vi "Actor Core.vi"(8 "error in":errorcluster, 11 "Preview in":refnum<class "Preview.lvclass">) -> (0 "error out":errorcluster, 3 "Actor out":refnum<class "Actor.lvclass">)   [LabVIEW 2018, in "Preview Window.lvlib" / "Preview.lvclass"]
doc: "(<B>Filename</B>: Actor Framework.lvlib:Actor.lvclass:Actor Core.vi)\n\nReceives messages to the actor, reacts to them, and initiates any error handling that may shut the actor down.\n\nDescendant classes may override this VI to append parallel tasks for the actor to complete while it handles messages. Overrides use the Call Parent Method node."
uses:
  Preview.lvclass
  C:/Users/Jeff Tipps/Documents/DAQMan/source/Classes/Actor Nest/Class Actor Nest/Actor Nest.lvclass
  C:/Program Files (x86)/National Instruments/LabVIEW 2018/vi.lib/ActorFramework/Actor/Actor.lvclass
  <vilib>/ActorFramework/Actor/Actor.lvclass
  Actor Nest/Class Actor Nest/Actor Nest.lvclass/Actor Nest.ctl
  <vilib>/ActorFramework/Actor/Actor.lvclass/Actor.ctl
  <vilib>/ActorFramework/Message Enqueuer/Message Enqueuer.lvclass/Message Enqueuer.ctl
  Actor Nest/Actor Nest Messages/Handle Nested Error Msg/Handle Nested Error Msg.lvclass/Handle Nested Error Msg.ctl
  Actor Nest/Class Actor Nest/Read Shutdown.vi
  <vilib>/ActorFramework/Message Enqueuer/Init from Existing Queue.vi
  <vilib>/ActorFramework/Message Enqueuer/Enqueue.vi
  Actor Nest/Actor Nest Messages/Handle Nested Error Msg/Handle Nested Error Msg.lvclass
  C:/Program Files (x86)/National Instruments/LabVIEW 2018/vi.lib/ActorFramework/Message/Message.lvclass
  <vilib>/ActorFramework/Stop Msg/Stop Msg.lvclass
  <vilib>/ActorFramework/Message Priority Queue/Priority Enqueue.vi
  <vilib>/ActorFramework/Message Enqueuer/Message Enqueuer.lvclass
  Actor Nest/Class Actor Nest/Actor Nest.lvclass
panel:
  in  "Stop Scalar":bool
  in  "Stop Wfm":bool
  in  "Legend LB":i32[](listbox)
  out "Wfm Graph":sgl[][](graph)
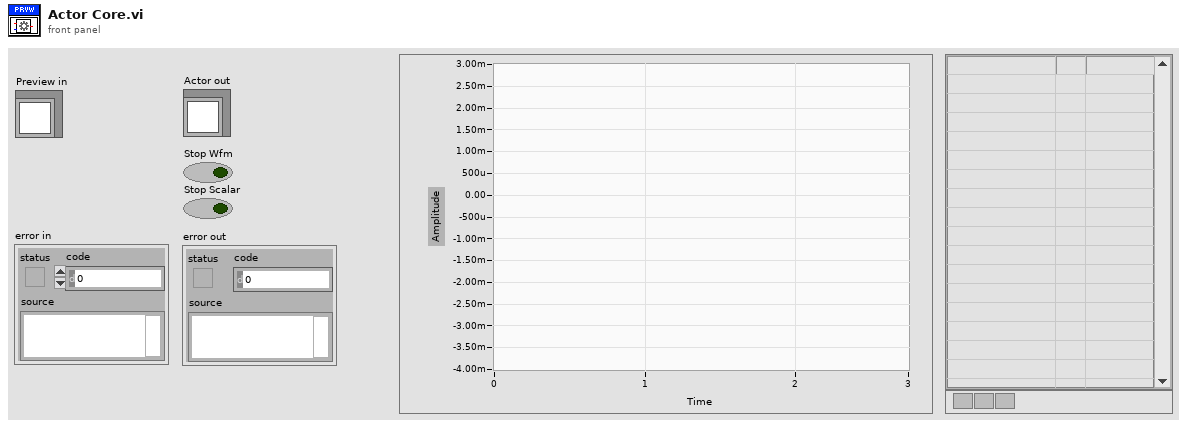
[diagram p1: front panel]
types:
  T1 = cluster{"Scalar Ntfr Name":string, "Num of Chans":i32, "Selected Chan Indeces":i32[]}
  T2 = cluster{"Wfm Ntfr Name":string, "Chart History":i32, "Selected Chan Indeces":i32[]}
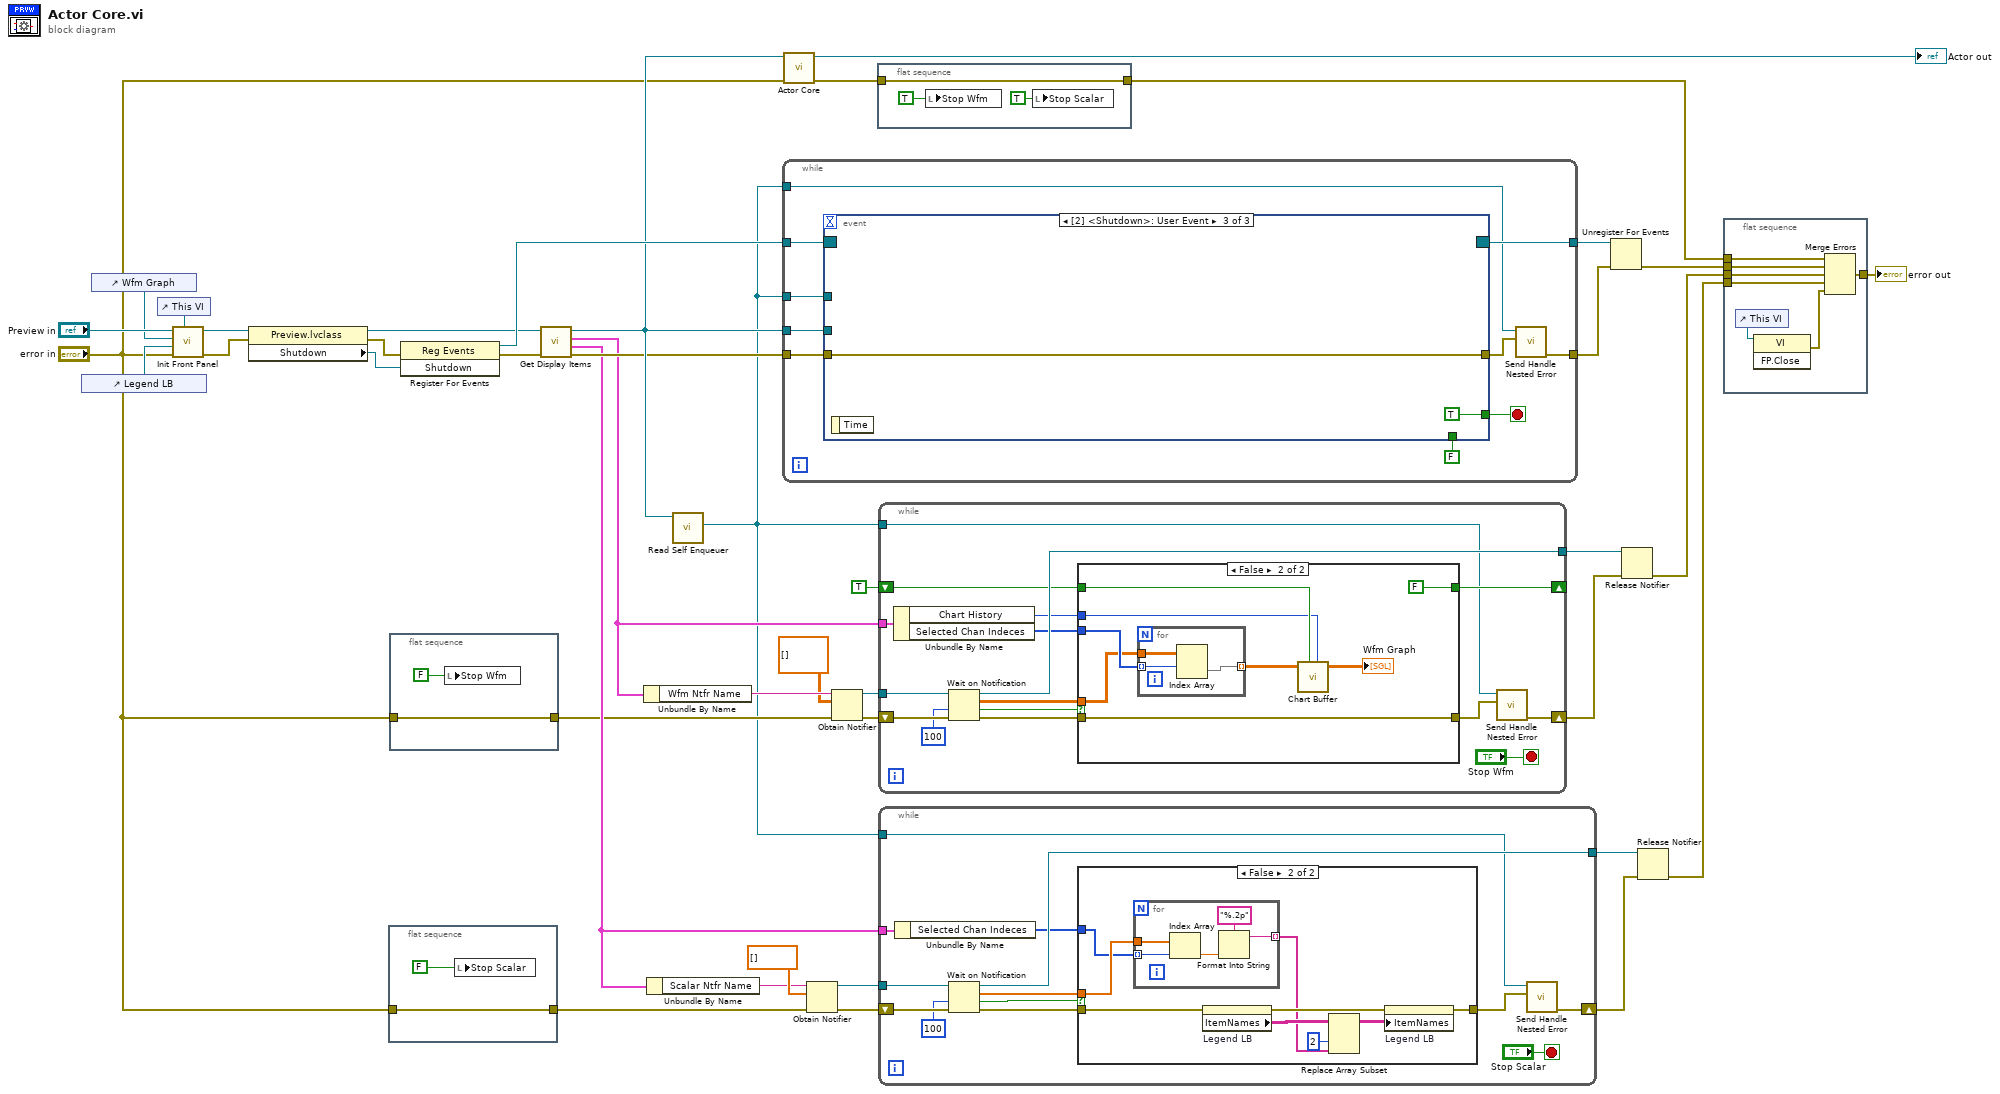
[diagram p0: block diagram]
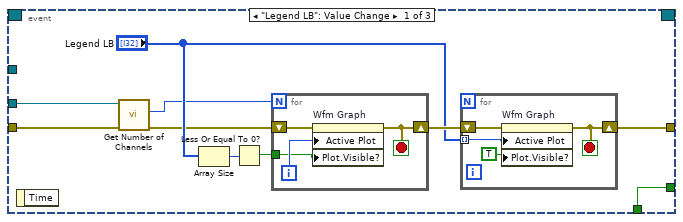
[diagram p4: hidden frame]
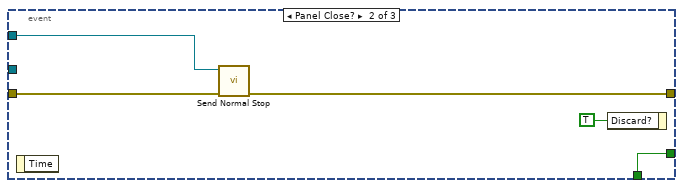
[diagram p5: hidden frame]
diagram:
  n1 = control-ref of="Legend LB"() -> (w40:refnum<vi>)
  n2 = control-ref of="Wfm Graph"() -> (w39:refnum<vi>)
  n3 = control-ref of="This VI"() -> (w38:refnum<vi>)
  n4 = call "Init Front Panel.vi"("This VI"=w38, "error in (no error)"="error in", "Legend LB"=w40, "Wfm Graph"=w39, "Preview in"="Preview in") -> ("error out"=w37:errorcluster, "Preview out"=w30:refnum<class "Preview.lvclass">)  [unwired: 5 in]
  n5 = property class="Preview.lvclass"(reference=w30, error in=w37) -> (reference out=w29:refnum<class "Preview.lvclass">, error out=w36:errorcluster, "Shutdown"=w35:refnum<user-event>)
  n6 = flat-sequence {
    tunnel: [w43] -> w5
    tunnel: "error in" -> [w43]
    frame #0 {
      n7 = local write "Stop Scalar"(FALSE ("Stop Wfm")) -> ()
    }
  }
  n8 = flat-sequence {
    tunnel: [w44] -> w11
    tunnel: "error in" -> [w44]
    frame #0 {
      n9 = local write "Stop Wfm"(FALSE ("Stop Wfm")) -> ()
    }
  }
  n10 = register-events(error in=w36, w35) -> (reference out=w34:refnum<event-registration>, error out=w28:errorcluster)  [unwired: 1 in]
  n11 = call "Get Display Items.vi"("error in (no error)"=w28, "Preview in"=w29) -> ("error out"=w26:errorcluster, "Scalar Items"=w12:T1, "Wfm Items"=w19:T2, "Preview out"=w27:refnum<class "Preview.lvclass">)  [unwired: 6 in]
  n12 = Unbundle By Name(w19) -> ("Wfm Ntfr Name"=w25:string)
  n13 = Unbundle By Name(w12) -> ("Scalar Ntfr Name"=w23:string)
  n14 = call <vilib>:"Read Self Enqueuer.vi"("Actor"=w27) -> ("Self Enqueuer"=w4:refnum<class "Message Enqueuer.lvclass">)  [unwired: 10 in]
  n15 = while {
    tunnel: w26 -> [w55]
    tunnel: w34 -> [w54]
    tunnel: [w53] -> w33
    tunnel: [w50] -> w32
    tunnel: w27 -> [w48]
    tunnel: w4 -> [w47]
    tunnel: w4 -> [w46]
    stop <- w52 stop-if-true
    n16 = event shown="[2] <Shutdown>: User Event" {
      selector: w54 -> [_ _ _]
      dyn-events: [_ _ _] -> w53
      timeout: _ -> [_ _ _]
      tunnel: w55 -> [w59 w76 w80]
      tunnel: [w65 w78 TRUE] -> w52
      tunnel: FALSE -> [w65 w78 _]
      tunnel: [w61 w75 w80] -> w49
      tunnel: w48 -> [w58 _ _]
      tunnel: w46 -> [_ w74 _]
      event "Legend LB": Value Change {
        n17 = event-data() -> ()  [unwired: 1 in, 1 out]
        n18 = call "Get Number of Channels.vi"("error in (no error)"=w59, "Preview in"=w58) -> ("error out"=w56:errorcluster, "size(s)"=w57:i32)  [unwired: 7 in, 1 out]
        n19 = Array Size(array="Legend LB") -> (size(s)=w62:i32)
        n20 = Less Or Equal To 0?(x=w62) -> (x <= 0?=w64:bool)
        n21 = for {
          N: w57 -> [_]
          tunnel: w64 -> [w66]
          shift-right: [w68] -> w63
          shift-left: w56 -> [w69]
          i -> [w67]
          stop <- w68 stop-if-true
          n22 = property on="Wfm Graph" class="WFGraph (strict)"(error in=w69, "Active Plot"=w67, "Plot.Visible?"=w66) -> (error out=w68:errorcluster)  [unwired: 1 in, 1 out]
        }
        n23 = for {
          tunnel: "Legend LB" -> [w72] mode=indexing
          shift-right: [w70] -> w61
          shift-left: w63 -> [w73]
          stop <- w70 stop-if-true
          n24 = property on="Wfm Graph" class="WFGraph (strict)"(error in=w73, "Active Plot"=w72, "Plot.Visible?"=TRUE ("Plot.Visible")) -> (error out=w70:errorcluster)  [unwired: 1 in, 1 out]
        }
      }
      event Panel Close? {
        n25 = event-data() -> ()  [unwired: 1 in, 1 out]
        n26 = call <vilib>:"Send Normal Stop.vi"("error in (no error)"=w76, "Message Enqueuer"=w74) -> ("error out"=w75:errorcluster)  [unwired: 9 in]
        n27 = event-data("Discard?"=TRUE) -> ()  [unwired: 1 in, 1 out]
      }
      event User Event {
        n28 = event-data() -> ()  [unwired: 1 in, 1 out]
      }
    }
    n29 = call "Send Handle Nested Error.vi"("Nested Error"=w49, "Message Enqueuer"=w47) -> ("error out"=w50:errorcluster)  [unwired: 8 in, 1 out]
  }
  n30 = call-parent "Actor Core.vi"("error in"="error in", "Actor in"=w27) -> ("error out"=w10:errorcluster, "Actor out"=→"Actor out":refnum<class "Actor.lvclass">)  [unwired: 8 in]
  n31 = Obtain Notifier(name (unnamed)=w23, notification data type=dbl[] [], error in (no error)=w5) -> (notifier out=w17:refnum<notifier>, error out=w18:errorcluster)  [unwired: 1 in, 1 out]
  n32 = Obtain Notifier(name (unnamed)=w25, notification data type=dbl[][] [], error in (no error)=w11) -> (notifier out=w22:refnum<notifier>, error out=w21:errorcluster)  [unwired: 1 in, 1 out]
  n33 = flat-sequence {
    tunnel: w10 -> [w83]
    tunnel: [w83] -> w3
    frame #0 {
      n34 = local write "Stop Wfm"(TRUE ("Stop Wfm")) -> ()
      n35 = local write "Stop Scalar"(TRUE ("Stop Scalar")) -> ()
    }
  }
  n36 = while {
    shift-right: [w86] -> w15
    shift-left: w21 -> [w98]
    tunnel: w22 -> [w99]
    tunnel: [w93] -> w16
    shift-right: [w91] -> _
    shift-left: TRUE -> [w92]
    tunnel: w19 -> [w88]
    tunnel: w4 -> [w84]
    stop <- "Stop Wfm" stop-if-true
    n37 = Unbundle By Name(w88) -> ("Chart History"=w90:i32, "Selected Chan Indeces"=w89:i32[])
    n38 = Wait on Notification(notifier=w99, timeout in ms (-1)=100, error in (no error)=w98) -> (notifier out=w93:refnum<notifier>, notification=w95:dbl[][], timed out?=w96:bool, error out=w97:errorcluster)  [unwired: 1 in]
    n39 = case shown="False" w96 {
      tunnel: w97 -> [w101 w109]
      tunnel: [w101 w109] -> w85
      tunnel: w89 -> [_ w108]
      tunnel: w95 -> [_ w107]
      tunnel: w92 -> [w100 w105]
      tunnel: [w100 FALSE] -> w91
      tunnel: w90 -> [_ w103]
      frame True {
      }
      frame False {
        n40 = for {
          tunnel: w108 -> [w112] mode=indexing
          tunnel: w107 -> [w111]
          tunnel: [w110] -> w106 mode=indexing
          n41 = Index Array(array=w111, index (row)=w112) -> (element=w110:dbl[])  [unwired: 1 in]
        }
        n42 = call "Chart Buffer.vi"("Wfm In"=w106, "Reset?"=w105, "Chart History"=w103) -> ("Wfm Out"=→"Wfm Graph":sgl[][])  [unwired: 6 in]
      }
    }
    n43 = call "Send Handle Nested Error.vi"("Nested Error"=w85, "Message Enqueuer"=w84) -> ("error out"=w86:errorcluster)  [unwired: 8 in, 1 out]
  }
  n44 = while {
    shift-right: [w116] -> w13
    shift-left: w18 -> [w124]
    tunnel: w17 -> [w125]
    tunnel: [w119] -> w14
    tunnel: w12 -> [w117]
    tunnel: w4 -> [w114]
    stop <- "Stop Scalar" stop-if-true
    n45 = Unbundle By Name(w117) -> ("Selected Chan Indeces"=w113:i32[])
    n46 = Wait on Notification(notifier=w125, timeout in ms (-1)=100, error in (no error)=w124) -> (notifier out=w119:refnum<notifier>, notification=w121:dbl[], timed out?=w122:bool, error out=w123:errorcluster)  [unwired: 1 in]
    n47 = case shown="False" w122 {
      tunnel: w123 -> [w126 w134]
      tunnel: [w126 w129] -> w115
      tunnel: w121 -> [_ w135]
      tunnel: w113 -> [_ w128]
      frame True {
      }
      frame False {
        n48 = for {
          tunnel: w135 -> [w139]
          tunnel: w128 -> [w138] mode=indexing
          tunnel: [w136] -> w127 mode=indexing
          n49 = Index Array(array=w139, index=w138) -> (element=w137:dbl)
          n50 = Format Into String(format string="%.2p", w137) -> (resulting string=w136:string)  [unwired: 2 in, 1 out]
        }
        n51 = property on="Legend LB" class="MCListbox (strict)"(error in=w134) -> (error out=w131:errorcluster, "ItemNames"=w133:string[][])  [unwired: 1 in, 1 out]
        n52 = Replace Array Subset(array=w133, new element=w127, index (col)=2 ("disabled index (col)")) -> (w130:string[][])  [unwired: 1 in]
        n53 = property on="Legend LB" class="MCListbox (strict)"(error in=w131, "ItemNames"=w130) -> (error out=w129:errorcluster)  [unwired: 1 in, 1 out]
      }
    }
    n54 = call "Send Handle Nested Error.vi"("Nested Error"=w115, "Message Enqueuer"=w114) -> ("error out"=w116:errorcluster)  [unwired: 8 in, 1 out]
  }
  n55 = Unregister For Events(event registration refnum=w33, error in=w32) -> (error out=w2:errorcluster)
  n56 = Release Notifier(notifier=w16, error in (no error)=w15) -> (error out=w9:errorcluster)  [unwired: 1 in, 2 out]
  n57 = Release Notifier(notifier=w14, error in (no error)=w13) -> (error out=w7:errorcluster)  [unwired: 1 in, 2 out]
  n58 = flat-sequence {
    tunnel: [w147] -> w31
    tunnel: w9 -> [w146]
    tunnel: w7 -> [w145]
    tunnel: w3 -> [w144]
    tunnel: w2 -> [w143]
    frame #0 {
      n59 = control-ref of="This VI"() -> (w141:refnum<vi>)
      n60 = invoke class="VI" method="FP.Close"(reference=w141) -> (error out=w142:errorcluster)  [unwired: 2 in, 2 out]
      n61 = Merge Errors(w144, w143, w146, w145, w142) -> (w147:errorcluster)
    }
  }
  "error out" <- w31
